vi "Append Composition.vi"(9 "Class":string, 10 "Private Data Control":refnum<vi>, 11 "Class Relations Map":T1(c390)) -> (3 "Class Relations Map Out":T1(c390))   [LabVIEW 2019]
uses:
  <vilib>/Utility/traverseref.llb/TRef TravTarget.ctl
  <vilib>/Utility/miscctls.llb/LVMapReplaceAction.ctl
  <vilib>/Utility/traverseref.llb/VI Scripting - Traverse.lvlib
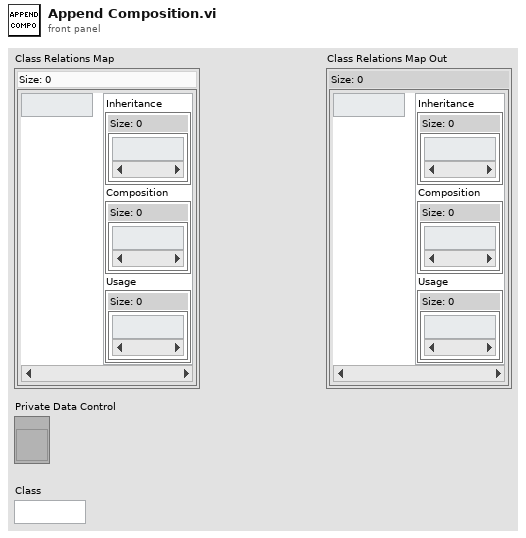
[diagram p1: front panel]
types:
  T1 = map{string, cluster{"Inheritance":set{string}, "Composition":set{string}, "Usage":set{string}}}
  T2 = typedef "TRef TravTarget.ctl" = enum16{"FP", "BD", "Other"}
  T3 = typedef "LVMapReplaceAction.ctl" = enum32{"Modify Entry only if found", "Add or Modify Entry", "Delete Entry"}
  T4 = cluster{"Inheritance":set{string}, "Composition":set{string}, "Usage":set{string}}
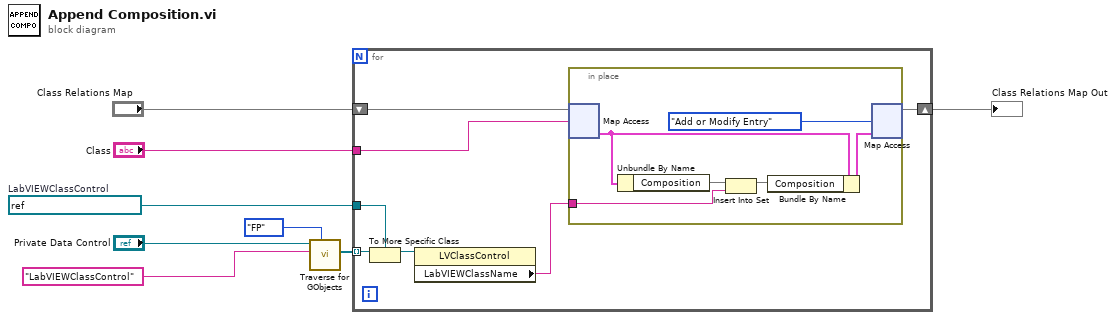
[diagram p0: block diagram]
diagram:
  w7 = refnum<vi> refnum  # LabVIEWClassControl
  n1 = call <vilib>:"Traverse for GObjects.vi"("Traverse Target"=TRef_TravTarget."FP", "Class Name"="LabVIEWClassControl", "VI Refnum"="Private Data Control") -> ("References"=w2:refnum<vi>[])  [unwired: 5 in, 3 out]
  n2 = for {
    tunnel: w2 -> [w15] mode=indexing
    tunnel: w7 -> [w13]
    shift-right: [w10] -> w3
    shift-left: "Class Relations Map" -> [w12]
    tunnel: "Class" -> [w9]
    n3 = To More Specific Class(target class=w13, reference=w15) -> (specific class reference=w14:refnum<vi>)  [unwired: 1 in, 1 out]
    n4 = property class="LVClassControl"(reference=w14) -> ("LabVIEWClassName"=w11:string)  [unwired: 1 in, 2 out]
    n5 = in-place {
      in-place-border: w11 -> [w19]
      n6 = in-place-map #1(w12, w9) -> (w18:T4)  [unwired: 1 in, 1 out]
      n7 = Unbundle By Name(w18) -> ("Composition"=w17:set{string})
      n8 = Insert Into Set(10:w19, 11:w17) -> (3:w20:set{string})  [unwired: 1 out]
      n9 = Bundle By Name(cluster=w18, "Composition"=w20) -> (w16:T4)
      n10 = in-place-map #1(w16, LVMapReplaceAction."Add or Modify Entry" ("action")) -> (w10:T1)  [unwired: 2 out]
    }
  }
  "Class Relations Map Out" <- w3
